vi "set_calcset.vi"(8 "error in":errorcluster, 11 "Calculation Settings":T1={"Verbose"=FALSE, "Uncertainty Calculation Method"=enum."None", "MCM Repeats"=1, "MCM Verbose"=FALSE, "MCM Calculation Method"=enum."Single Core", "MCM Processes"=1, "MCM Temporary Dir"=path ""} {"MCM Processes" min=1 step=1; "MCM Repeats" min=1 step=1}) -> (0 "error out":errorcluster)   [LabVIEW 2013]
uses:
  TD Calculation Settings.ctl
  TD Uncertainty Calculation Method.ctl
  TD MCM Calculation Method.ctl
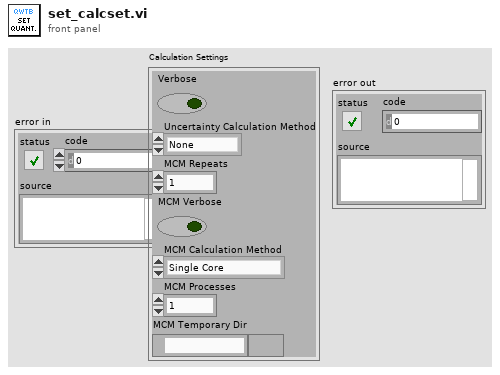
[diagram p1: front panel]
types:
  T1 = typedef "TD Calculation Settings.ctl" = cluster{"Verbose":bool, "Uncertainty Calculation Method":T2, "MCM Repeats":i32, "MCM Verbose":bool, "MCM Calculation Method":T3, "MCM Processes":i32, "MCM Temporary Dir":path}
  T2 = typedef "TD Uncertainty Calculation Method.ctl" = enum16{"None", "GUF", "MCM"}
  T3 = typedef "TD MCM Calculation Method.ctl" = enum16{"Single Core", "Single Station", "Multi Station"}
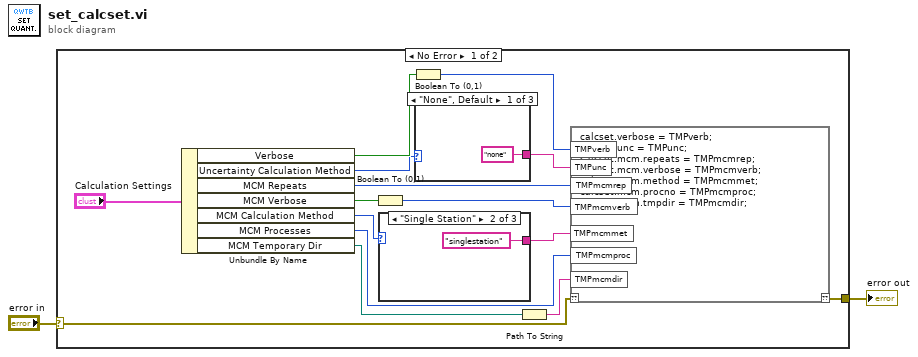
[diagram p0: block diagram]
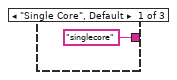
[diagram p2: hidden frame]
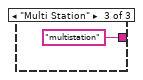
[diagram p3: hidden frame]
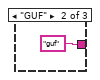
[diagram p4: hidden frame]
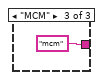
[diagram p5: hidden frame]
diagram:
  n1 = case shown="No Error" "error in" {
    selector: "error in" -> [w4 w24]
    tunnel: [w17 w24] -> w2
    frame No Error {
      n2 = Unbundle By Name("Calculation Settings") -> ("Verbose"=w15:bool, "Uncertainty Calculation Method"=w12:T2, "MCM Repeats"=w9:i32, "MCM Verbose"=w13:bool, "MCM Calculation Method"=w10:T3, "MCM Processes"=w7:i32, "MCM Temporary Dir"=w5:path)
      n3 = Boolean To (0,1)(Boolean=w13) -> (0, 1=w14:i16)
      n4 = case shown="\"Single Station\"" w10 {
        tunnel: ["singlecore" ("String") "singlestation" ("String") "multistation" ("String")] -> w8
        frame "Single Core", Default {
        }
        frame "Single Station" {
        }
        frame "Multi Station" {
        }
      }
      n5 = Boolean To (0,1)(Boolean=w15) -> (0, 1=w16:i16)
      n6 = case shown="\"None\", Default" w12 {
        tunnel: ["none" ("String") "guf" ("String") "mcm" ("String")] -> w11
        frame "None", Default {
        }
        frame "GUF" {
        }
        frame "MCM" {
        }
      }
      n7 = Path To String(path=w5) -> (string=w6:string)
      n8 = script code="calcset.verbose = TMPverb;\ncalcset.unc = TMPunc;\ncalcset.mcm.repeats = TMPmcmrep;\ncalcset.mcm.verbose = TMPmcmverb;\ncalcset.mcm.method = TMPmcmmet;\ncalcset.mcm.procno = TMPmcmproc;\ncalcset.mcm.tmpdir = TMPmcmdir;"("??"=w4, "TMPverb"=w16, "TMPunc"=w11, "TMPmcmrep"=w9, "TMPmcmverb"=w14, "TMPmcmmet"=w8, "TMPmcmproc"=w7, "TMPmcmdir"=w6) -> ("??"=w17:errorcluster)
    }
    frame Error {
    }
  }
  "error out" <- w2
